vi "SCOnly2.vi"() -> ()   [LabVIEW 2014]
uses:
  <vilib>/Instr/_visa.llb/VISA Configure Serial Port (Instr).vi
panel:
  in  "Si Speed Ctrl":i32=2000
  in  "Si Mid":i32=26000
  in  "Si In":i32=49000
  in  "TLSpeedCtrl":i32=4000
  in  "Pos5":i32=429000
  in  "Pos4":i32=339000
  in  "Pos3":i32=249000
  in  "Pos2":i32=163000
  in  "Pos1":i32=71000
  in  "Main SC Loop":bool
  out "Position1":i32 min=0 format="%#.10f"
  out "Position2":i32 min=0 format="%#.10f"
  out "Position3":i32 min=0 format="%#.10f"
  out "Position4":i32 min=0 format="%#.10f"
  out "Position5":i32 min=0 format="%#.10f"
  out "TL Speed":i32 min=0 format="%#.10f"
  out "Si IN":i32 min=0 format="%#.10f"
  out "Si Speed":i32 min=0 format="%#.10f"
  out "Si MID":i32 min=0 format="%#.10f"
  in  "Pos1 Enable":bool=TRUE
  in  "Pos2 Enable":bool=TRUE
  in  "Pos3 Enable":bool=TRUE
  in  "Pos4 Enable":bool=TRUE
  in  "Pos5 Enable":bool=TRUE
  in  "TL":T1(radio)=enum."Radio Selection 1"
  in  "Normal/Overide":bool=TRUE
  out "TL Input":string
  out "TL Output":string
  out "Si Input":string
  out "Si Output":string
  out "TL in Position?":bool=TRUE
  out "Si in Position?":bool=TRUE
  in  "TL Test":bool=TRUE
  in  "Si Test":bool=TRUE
  out "Tl Test Readout":string
  out "Si Test Readout":string
  out "Tl Test String":string
  out "Si Test String":string
  in  "TL Test Steps":dbl format="%#_13g"
  in  "Si Test Steps":dbl format="%#_13g"
  out "Si Abort Readout":string
  out "TL Abort readout":string
  in  "Abort SC":bool=TRUE
  in  "Si":T2(radio)=enum."Radio Selection 1"
  out "Si Position":i32
  out "Si Bar":i32(slide) scale=0.0..49001.0
  out "TL Position":i32
  out "TL Bar":i32(slide) scale=0.0..429000.0
  in  "SC On/Off":bool
  out "TL Position Readout":string
  out "Si Position Readout":string
  # "Faraday Cup"
  # "Si Home"
  # "Testing/Manual"
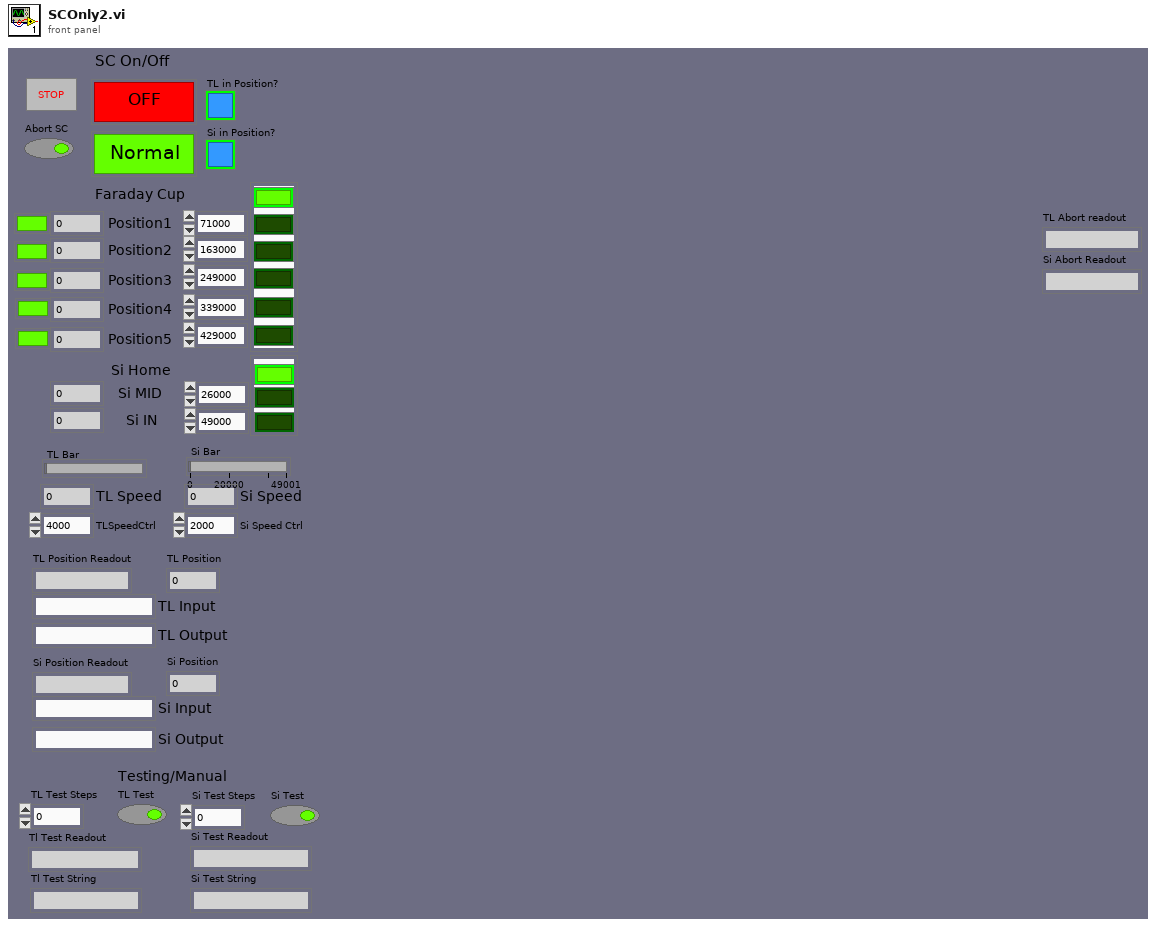
[diagram p1: front panel]
types:
  T1 = enum32{"No Selection", "Radio Selection 1", "Radio Selection 2", "Radio Selection 3", "Radio Selection 4", "Radio Selection 5", "Radio Selection 6"}
  T2 = enum32{"No Selection", "Radio Selection 1", "Radio Selection 2", "Radio Selection 3"}
  T3 = cluster{"read buffer":string, "Numeric":i32, "read buffer":string, "Numeric":i32, bool}
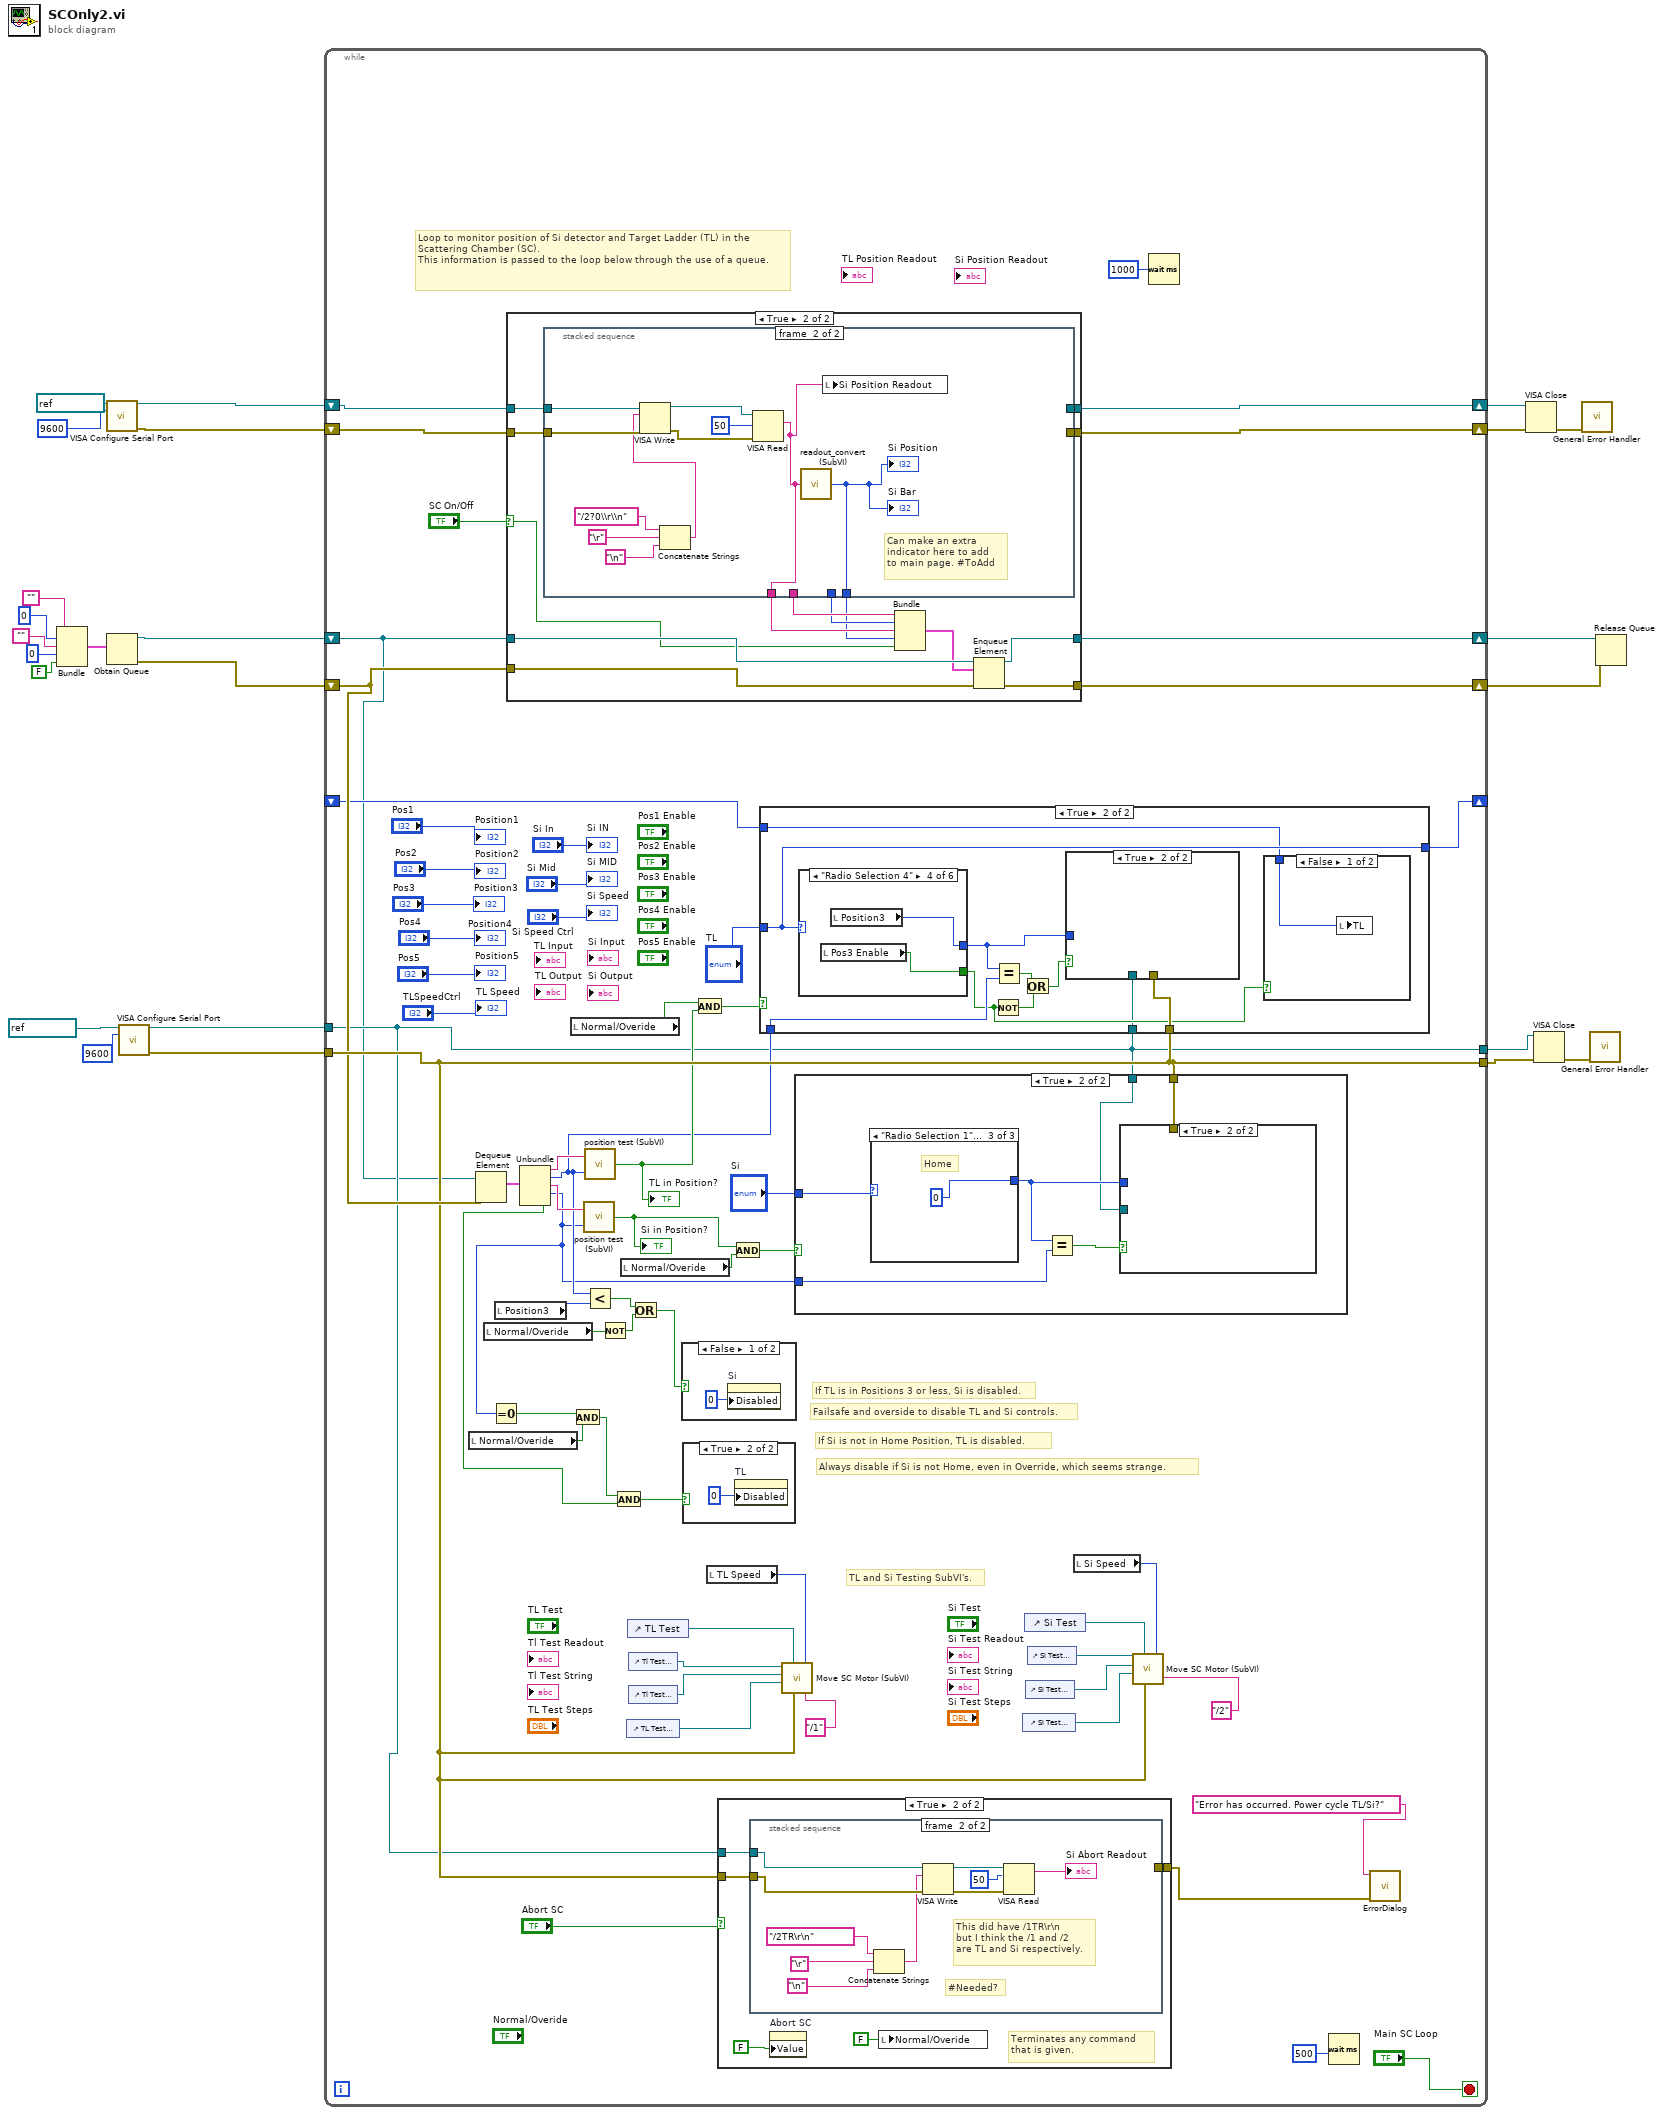
[diagram p0: block diagram]
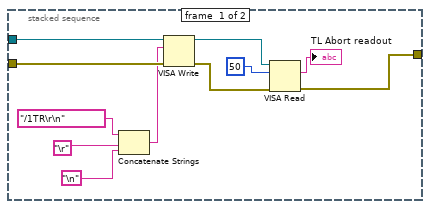
[diagram p3: hidden frame]
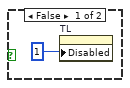
[diagram p4: hidden frame]
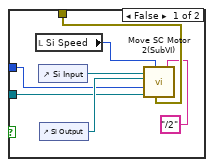
[diagram p6: hidden frame]
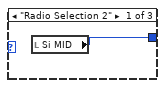
[diagram p7: hidden frame]
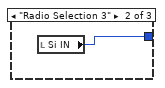
[diagram p8: hidden frame]
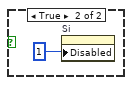
[diagram p9: hidden frame]
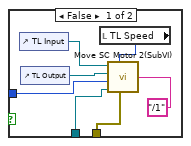
[diagram p12: hidden frame]
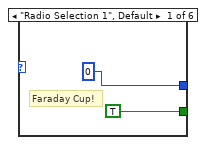
[diagram p13: hidden frame]
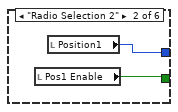
[diagram p14: hidden frame]
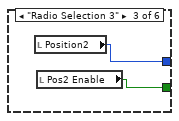
[diagram p15: hidden frame]
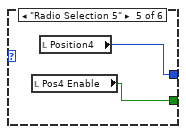
[diagram p16: hidden frame]
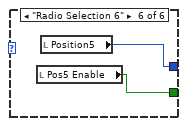
[diagram p17: hidden frame]
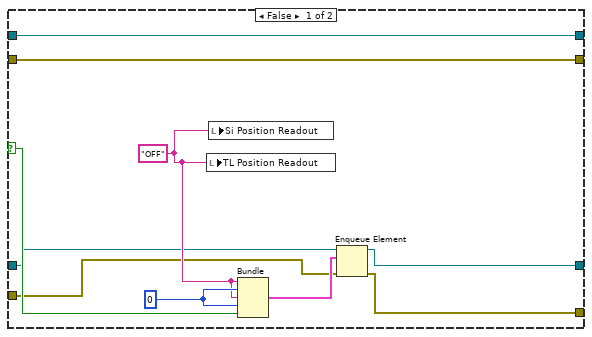
[diagram p18: hidden frame]
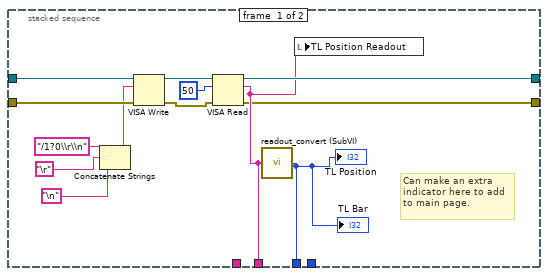
[diagram p19: hidden frame]
diagram:
  n1 = Bundle("", 0, "", 0, FALSE) -> (w16:cluster{string, i32, string, i32, bool})  [unwired: 1 in]
  n2 = call-poly "VISA Configure Serial Port"("VISA resource name"=refnum<visa-resource-name> "COM29" ("Resource Name"), "baud rate (9600)"=u32 9600 ("Baud Rate (9600)")) -> ("VISA resource name out"=w15:refnum<visa-resource-name>, "error out"=w14:errorcluster)  [unwired: 12 in]
  n3 = Obtain Queue(element data type=w16) -> (queue out=w6:refnum<queue>, error out=w5:errorcluster)  [unwired: 4 in, 1 out]
  n4 = call-poly "VISA Configure Serial Port"("VISA resource name"=refnum<visa-resource-name> "COM29" ("Resource Name"), "baud rate (9600)"=u32 9600 ("Baud Rate (9600)")) -> ("VISA resource name out"=w1:refnum<visa-resource-name>, "error out"=w3:errorcluster)  [unwired: 12 in]
  n5 = while {
    tunnel: w3 -> [w26]
    shift-right: [w83] -> w11
    shift-left: w15 -> [w86]
    shift-right: [w84] -> w13
    shift-left: w14 -> [w85]
    shift-right: [w81] -> w9
    shift-left: w6 -> [w24]
    shift-right: [w82] -> w10
    shift-left: w5 -> [w80]
    shift-right: [w27] -> _
    shift-left: _ -> [w28]
    tunnel: [w26] -> _
    tunnel: [w25] -> w2
    tunnel: w1 -> [w25]
    stop <- "Main SC Loop" stop-if-true
    # "Always disable if Si is not Home, even in Override, which seems strange."
    # "TL and Si Testing SubVI's."
    # "If Si is not in Home Position, TL is disabled."
    # "If TL is in Positions 3 or less, Si is disabled."
    # "Failsafe and overside to disable TL and Si controls."
    # "Loop to monitor position of Si detector and Target Ladder (TL) in the Scattering Chamber (SC). \nThis information is passed to the loop below through the use of a queue."
    n6 = local read "Normal/Overide"() -> (w52:bool)
    n7 = Dequeue Element(queue=w24, error in (no error)=w80) -> (element=w66:cluster{string, i32, string, i32, bool})  [unwired: 1 in, 3 out]
    n8 = local read "Normal/Overide"() -> (w33:bool)
    n9 = local read "Position3"() -> (w59:i32)
    n10 = case shown="True" "SC On/Off" {
      selector: "SC On/Off" -> [w170 w186]
      tunnel: w80 -> [w167 w188]
      tunnel: w24 -> [w168 w187]
      tunnel: w86 -> [w174 w185]
      tunnel: w85 -> [w173 w184]
      tunnel: [w173 w183] -> w84
      tunnel: [w174 w182] -> w83
      tunnel: [w166 w176] -> w82
      tunnel: [w165 w175] -> w81
      frame False {
        w171 = "OFF"
        w172 = 0
        n11 = local write "TL Position Readout"(w171) -> ()
        n12 = local write "Si Position Readout"(w171) -> ()
        n13 = Bundle(w171, w172, w171, w172, w170) -> (w169:cluster{string, i32, string, i32, bool})  [unwired: 1 in]
        n14 = Enqueue Element(queue=w168, element=w169, error in (no error)=w167) -> (queue out=w165:refnum<queue>, error out=w166:errorcluster)  [unwired: 1 in, 1 out]
      }
      frame True {
        n15 = stacked-sequence {
          tunnel: w185 -> [w201 w209]
          tunnel: w184 -> [w200 w208]
          tunnel: [w189 _] -> w183
          tunnel: [w193 _] -> w182
          tunnel: [w192 _] -> w181
          tunnel: [w190 _] -> w180
          tunnel: [_ w203] -> w179
          tunnel: [_ w202] -> w178
          frame #0 {
            # "Can make an extra \nindicator here to add\nto main page."
            n16 = Concatenate Strings("/1?0\\r\\n", "\r", "\n") -> (w196:string)
            n17 = VISA Write(VISA resource name=w201, write buffer=w196, error in (no error)=w200) -> (VISA resource name out=w195:refnum<visa-resource-name>, error out=w194:errorcluster)  [unwired: 1 out]
            n18 = VISA Read(VISA resource name=w195, byte count=50, error in (no error)=w194) -> (VISA resource name out=w193:refnum<visa-resource-name>, read buffer=w192:string, error out=w189:errorcluster)  [unwired: 1 out]
            n19 = call "readout_convert (SubVI).vi"("read buffer"=w192) -> ("Numeric"=w190:i32)
            "TL Position" <- w190
            "TL Bar" <- w190
            n20 = local write "TL Position Readout"(w192) -> ()
          }
          frame #1 {
            # "Can make an extra \nindicator here to add\nto main page. #ToAdd"
            n21 = Concatenate Strings("/2?0\\r\\n", "\r", "\n") -> (w204:string)
            n22 = VISA Write(VISA resource name=w209, write buffer=w204, error in (no error)=w208) -> (VISA resource name out=w205:refnum<visa-resource-name>, error out=w207:errorcluster)  [unwired: 1 out]
            n23 = VISA Read(VISA resource name=w205, byte count=50, error in (no error)=w207) -> (read buffer=w203:string)  [unwired: 3 out]
            n24 = call "readout_convert (SubVI).vi"("read buffer"=w203) -> ("Numeric"=w202:i32)
            "Si Position" <- w202
            "Si Bar" <- w202
            n25 = local write "Si Position Readout"(w203) -> ()
          }
        }
        n26 = Bundle("read buffer"=w181, "Numeric"=w180, "read buffer"=w179, "Numeric"=w178, w186) -> (w177:T3)  [unwired: 1 in]
        n27 = Enqueue Element(queue=w187, element=w177, error in (no error)=w188) -> (queue out=w175:refnum<queue>, error out=w176:errorcluster)  [unwired: 1 in, 1 out]
      }
    }
    n28 = Unbundle(w66) -> (w65:string, w60:i32, w64:string, w34:i32, w49:bool)
    n29 = Equal To 0?(x=w34) -> (x = 0?=w53:bool)
    n30 = local read "Normal/Overide"() -> (w63:bool)
    n31 = And(x=w53, y=w52) -> (x .and. y?=w50:bool)
    n32 = call "position test (SubVI).vi"("Numeric"=w34, "String"=w64) -> ("Boolean"=w55:bool)
    "Si in Position?" <- w55
    n33 = call "position test (SubVI).vi"("Numeric"=w60, "String"=w65) -> ("Boolean"=w61:bool)
    "TL in Position?" <- w61
    n34 = Less?(x=w60, y=w59) -> (x < y?=w58:bool)
    n35 = Not(x=w33) -> (.not. x?=w32:bool)
    n36 = And(x=w50, y=w49) -> (x .and. y?=w51:bool)
    n37 = local read "Normal/Overide"() -> (w56:bool)
    n38 = control-ref of="TL Test Steps"() -> (w44:refnum<vi>)
    n39 = control-ref of="TL Test"() -> (w47:refnum<vi>)
    n40 = control-ref of="Tl Test Readout"() -> (w46:refnum<vi>)
    n41 = control-ref of="Tl Test String"() -> (w45:refnum<vi>)
    n42 = Or(x=w58, y=w32) -> (x .or. y?=w57:bool)
    n43 = case shown="False" w57 {
      frame False {
        n44 = property on="Si" class="RadioBtnsControl (strict)"("Disabled"=0) -> ()  [unwired: 2 in, 2 out]
      }
      frame True {
        n45 = property on="Si" class="RadioBtnsControl (strict)"("Disabled"=1) -> ()  [unwired: 2 in, 2 out]
      }
    }
    n46 = case shown="True" w51 {
      frame False {
        n47 = property on="TL" class="RadioBtnsControl (strict)"("Disabled"=1) -> ()  [unwired: 2 in, 2 out]
      }
      frame True {
        n48 = property on="TL" class="RadioBtnsControl (strict)"("Disabled"=0) -> ()  [unwired: 2 in, 2 out]
      }
    }
    n49 = And(x=w63, y=w61) -> (x .and. y?=w62:bool)
    n50 = local read "TL Speed"() -> (w48:i32)
    n51 = case shown="True" "Abort SC" {
      tunnel: w26 -> [w87 w92]
      tunnel: [w87 w89] -> w31
      tunnel: w25 -> [_ w88]
      frame False {
      }
      frame True {
        # "Terminates any command \nthat is given."
        n52 = stacked-sequence {
          tunnel: w92 -> [w103 w113]
          tunnel: [w94 _] -> w89
          tunnel: w88 -> [w93 w104]
          frame #0 {
            n53 = Concatenate Strings("/1TR\r\n", "\r", "\n") -> (w96:string)
            n54 = VISA Write(VISA resource name=w93, write buffer=w96, error in (no error)=w103) -> (VISA resource name out=w101:refnum<visa-resource-name>, error out=w102:errorcluster)  [unwired: 1 out]
            n55 = VISA Read(VISA resource name=w101, byte count=u32 50, error in (no error)=w102) -> (read buffer=→"TL Abort readout":string, error out=w94:errorcluster)  [unwired: 2 out]
          }
          frame #1 {
            # "#Needed?"
            # "This did have /1TR\\r\\n \nbut I think the /1 and /2 \nare TL and Si respectively."
            n56 = Concatenate Strings("/2TR\r\n", "\r", "\n") -> (w108:string)
            n57 = VISA Write(VISA resource name=w104, write buffer=w108, error in (no error)=w113) -> (VISA resource name out=w107:refnum<visa-resource-name>, error out=w106:errorcluster)  [unwired: 1 out]
            n58 = VISA Read(VISA resource name=w107, byte count=u32 50, error in (no error)=w106) -> (read buffer=→"Si Abort Readout":string)  [unwired: 3 out]
          }
        }
        n59 = property on="Abort SC" class="Bool (strict)"("Value"=FALSE) -> ()  [unwired: 2 in, 2 out]
        n60 = local write "Normal/Overide"(FALSE) -> ()
      }
    }
    n61 = And(x=w55, y=w56) -> (x .and. y?=w54:bool)
    n62 = case shown="True" w62 {
      tunnel: "TL" -> [w134 w137]
      tunnel: w60 -> [_ w141]
      tunnel: w26 -> [_ w139]
      tunnel: [w134 w137] -> w27
      tunnel: w28 -> [_ w136]
      tunnel: w25 -> [_ w135]
      frame False {
      }
      frame True {
        n63 = case shown="\"Radio Selection 4\"" w137 {
          tunnel: [0 w156 w158 w160 w162 w164] -> w142
          tunnel: [TRUE w155 w157 w159 w161 w163] -> w138
          frame "Radio Selection 1", Default {
            # "Faraday Cup!"
          }
          frame "Radio Selection 2" {
            n64 = local read "Pos1 Enable"() -> (w155:bool)
            n65 = local read "Position1"() -> (w156:i32)
          }
          frame "Radio Selection 3" {
            n66 = local read "Position2"() -> (w158:i32)
            n67 = local read "Pos2 Enable"() -> (w157:bool)
          }
          frame "Radio Selection 4" {
            n68 = local read "Pos3 Enable"() -> (w159:bool)
            n69 = local read "Position3"() -> (w160:i32)
          }
          frame "Radio Selection 5" {
            n70 = local read "Pos4 Enable"() -> (w161:bool)
            n71 = local read "Position4"() -> (w162:i32)
          }
          frame "Radio Selection 6" {
            n72 = local read "Pos5 Enable"() -> (w163:bool)
            n73 = local read "Position5"() -> (w164:i32)
          }
        }
        n74 = Not(x=w138) -> (.not. x?=w143:bool)
        n75 = Equal?(x=w142, y=w141) -> (x = y?=w144:bool)
        n76 = Or(x=w144, y=w143) -> (x .or. y?=w140:bool)
        n77 = case shown="True" w140 {
          tunnel: w142 -> [w149 _]
          tunnel: w139 -> [w148 _]
          tunnel: w135 -> [w146 _]
          frame False {
            n78 = control-ref of="TL Input"() -> (w151:refnum<vi>)
            n79 = control-ref of="TL Output"() -> (w150:refnum<vi>)
            n80 = local read "TL Speed"() -> (w152:i32)
            n81 = call "Move SC Motor 2(SubVI).vi"("String"="/1", "error out"=w148, "Speed"=w152, "VISA resource name out"=w146, "Position"=w149, "Output"=w150, "Input"=w151) -> ()
          }
          frame True {
          }
        }
        n82 = case shown="False" w138 {
          tunnel: w136 -> [w145 _]
          frame False {
            n83 = local write "TL"(w145) -> ()
          }
          frame True {
          }
        }
      }
    }
    n84 = call "Move SC Motor (SubVI).vi"("String"="/1", "Speed"=w48, "error out"=w26, "Button"=w47, "Steps"=w44, "Output"=w45, "Input"=w46) -> ()  [unwired: 1 in]
    n85 = case shown="True" w54 {
      tunnel: w34 -> [_ w120]
      tunnel: w26 -> [_ w118]
      tunnel: "Si" -> [_ w117]
      tunnel: w25 -> [_ w116]
      frame False {
      }
      frame True {
        n86 = case shown="\"Radio Selection 1\", Default" w117 {
          tunnel: [w129 w130 0] -> w121
          frame "Radio Selection 2" {
            n87 = local read "Si MID"() -> (w129:i32)
          }
          frame "Radio Selection 3" {
            n88 = local read "Si IN"() -> (w130:i32)
          }
          frame "Radio Selection 1", Default {
            # "Home"
          }
        }
        n89 = Equal?(x=w121, y=w120) -> (x = y?=w119:bool)
        n90 = case shown="True" w119 {
          tunnel: w121 -> [w124 _]
          tunnel: w118 -> [w125 _]
          tunnel: w116 -> [w122 _]
          frame False {
            n91 = local read "Si Speed"() -> (w128:i32)
            n92 = control-ref of="Si Input"() -> (w127:refnum<vi>)
            n93 = control-ref of="Si Output"() -> (w126:refnum<vi>)
            n94 = call "Move SC Motor 2(SubVI).vi"("String"="/2", "error out"=w125, "Speed"=w128, "VISA resource name out"=w122, "Position"=w124, "Output"=w126, "Input"=w127) -> ()
          }
          frame True {
          }
        }
      }
    }
    n95 = control-ref of="Si Test Steps"() -> (w38:refnum<vi>)
    n96 = control-ref of="Si Test"() -> (w41:refnum<vi>)
    n97 = control-ref of="Si Test String"() -> (w39:refnum<vi>)
    n98 = control-ref of="Si Test Readout"() -> (w40:refnum<vi>)
    n99 = local read "Si Speed"() -> (w42:i32)
    n100 = call "Move SC Motor (SubVI).vi"("String"="/2", "Speed"=w42, "error out"=w26, "Button"=w41, "Steps"=w38, "Output"=w39, "Input"=w40) -> ()  [unwired: 1 in]
    n101 = Wait (ms)(milliseconds to wait=1000) -> ()  [unwired: 1 out]
    n102 = Wait (ms)(milliseconds to wait=500) -> ()  [unwired: 1 out]
    n103 = call "ErrorDialog.vi"("error in (no error)"=w31, "message"="Error has occurred. Power cycle TL/Si?") -> ()  [unwired: 10 in]
    "Position1" <- "Pos1"
    "Position2" <- "Pos2"
    "Position3" <- "Pos3"
    "Position4" <- "Pos4"
    "Position5" <- "Pos5"
    "TL Speed" <- "TLSpeedCtrl"
    "Si IN" <- "Si In"
    "Si Speed" <- "Si Speed Ctrl"
    "Si MID" <- "Si Mid"
  }
  n104 = VISA Close(VISA resource name=w11, error in (no error)=w13) -> (error out=w12:errorcluster)
  n105 = VISA Close(VISA resource name=w2, error in (no error)=w3) -> (error out=w4:errorcluster)
  n106 = call <vilib>:"General Error Handler.vi"("error in (no error)"=w12) -> ()  [unwired: 10 in, 5 out]
  n107 = call <vilib>:"General Error Handler.vi"("error in (no error)"=w4) -> ()  [unwired: 10 in, 5 out]
  n108 = Release Queue(queue=w9, error in (no error)=w10) -> ()  [unwired: 1 in, 3 out]
